vi "__uintSetTimeout.vi"(8 "Error in (no error)":errorcluster, 10 "Timeout (-1)":T1=-1, 11 "Uint in":refnum<class "UintClass.lvclass">) -> (0 "Error out":errorcluster, 3 "Uint out":refnum<class "UintClass.lvclass">)   [LabVIEW 2011, in "UintClass.lvclass"]
uses:
  UintClass.lvclass
  timeout.ctl
  UintClass.lvclass/UintClass.ctl
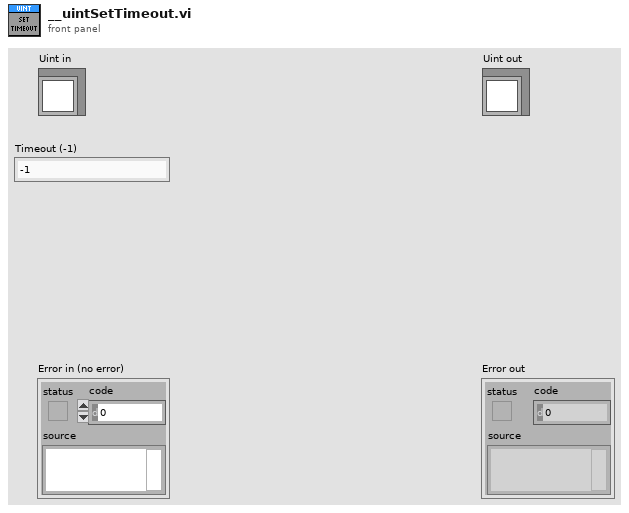
[diagram p1: front panel]
types:
  T1 = typedef "UintClass.lvclass/timeout.ctl" = i32
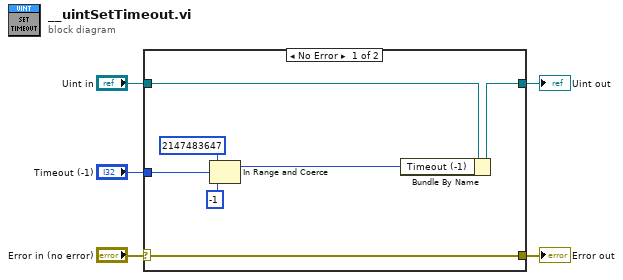
[diagram p0: block diagram]
diagram:
  n1 = case shown="No Error" "Error in (no error)" {
    selector: "Error in (no error)" -> [w12 w13]
    tunnel: [w12 w13] -> w4
    tunnel: [w10 w14] -> w2
    tunnel: "Uint in" -> [w11 w14]
    tunnel: "Timeout (-1)" -> [w9 _]
    frame No Error {
      n2 = In Range and Coerce(upper limit=T1 2147483647, x=w9, lower limit=T1 -1) -> (coerced(x)=w8:T1)  [unwired: 1 out]
      n3 = Bundle By Name(cluster=w11, "Timeout (-1)"=w8) -> (w10:refnum<class "UintClass.lvclass">)
    }
    frame Error {
    }
  }
  "Error out" <- w4
  "Uint out" <- w2
